vi "stabilizePress_00.vi"() -> ()   [LabVIEW 2011]
uses:
  <vilib>/Platform/TimedLoop/XDataNode/timing_clust.ctl
  <vilib>/Platform/TimedLoop/XDataNode/nitl_modes.ctl
  <vilib>/Platform/TimedLoop/XDataNode/wakeup.ctl
  <vilib>/Platform/TimedLoop/XDataNode/XDataNode.xnode
  <vilib>/Platform/TimedLoop/XDataNode/XDNodeRunTimeDep.lvlib
  <vilib>/Analysis/NI_AALPro.lvlib
panel:
  in  "local when done":bool=TRUE
  out "Best Exponential Fit":dbl[](array[numeric])=[19.840050765406623, 19.861458745604583, 19.86363222245769, 19.863852887909882, 19.863875291296292, 19.863877565833235, 19.86387779675896, 19.86387782020404, 19.86387782258433, 19.863877822825998, 19.863877822850533, 19.863877822853024]
  out "XY Graph":cluster{"Value":dbl[], "Value":dbl[]}[](graph)=[{"Value"=[1.0, 2.0, 3.0, 4.0, 5.0, 6.0, 7.0, 8.0, 9.0, 10.0, 11.0, 12.0], "Value"=[19.84, 19.86, 19.87, 19.87, 19.86, 19.86, 19.86, 19.87, 19.87, 19.86, 19.86, 19.86]}, {"Value"=[1.0, 2.0, 3.0, 4.0, 5.0, 6.0, 7.0, 8.0, 9.0, 10.0, 11.0, 12.0], "Value"=[19.840050765406623, 19.861458745604583, 19.86363222245769, 19.863852887909882, 19.863875291296292, 19.863877565833235, 19.86387779675896, 19.86387782020404, 19.86387782258433, 19.863877822825998, 19.863877822850533, 19.863877822853024]}]
  out "Pfinal (torr)":dbl=19.863877822853304
  out "tune done":bool=TRUE
  in  "max dP step (torr)":dbl=0.1
  out "dP(torr)":dbl
  out "amplitude":dbl=-0.23468810963673434
  out "damping":dbl=-2.287435637167759
  out "tune Setpoint(torr)":dbl=20.0
  in  "t array":dbl[](array[numeric])=[1.0, 2.0, 3.0, 4.0, 5.0, 6.0, 7.0, 8.0, 9.0, 10.0, 11.0, 12.0]
  out "P array":dbl[](array[numeric])=[19.84, 19.86, 19.87, 19.87, 19.86, 19.86, 19.86, 19.87, 19.87, 19.86, 19.86, 19.86]
  out "fit done":bool=TRUE
  in  "tFit(s)":dbl=10.0
  in  "Period (s)":i64=1
  out "Set Point (torr)":dbl=20.0 format="%.2f"
  out "Setpoint Index":string="C"
  out "Setpoint Index control":u16(ring)=2 caption="Setpoint" items=["A", "B", "C", "D"]
  out "first":bool
  out "tStart":dbl=12.0
  in  "time done (s)":dbl
  out "Wait to set":bool
  out "IO error":errorcluster
  in  "stop":bool
  out "P (torr)":dbl=19.86 format="%.2f"
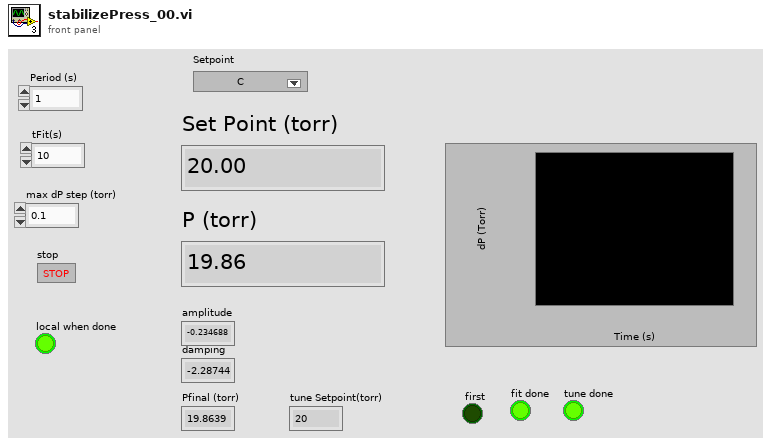
[diagram p1: front panel]
types:
  T1 = typedef "XDNodeRunTimeDep.lvlib/timing_clust.ctl" = cluster{"Expected End [f-1]":u64, "Actual End [f-1]":u64, "Finished Late? [f-1]":bool, "Expected End [i-1]":u64, "Actual End [i-1]":u64, "Finished Late? [i-1]":bool, "Expected Start [i]":u64, "Actual Start [i]":u64, "Expected Start [f]":u64, "Actual Start [f]":u64, "Source Name":string, "Structure Name":string, "Period":i64, "Deadline":i64, "Offset":i64, "Start":i64, "Priority":i32, "Timeout":i32, "Mode":T2, "Wakeup Reason":T3, "Error":errorcluster, "Source Type":string, "Secondary Source Type":string, "Global End Time":u64, "Global Start Time":u64, "Frame Duration":u64, "Iteration Duration":u64, "Assigned CPU":i32, "I/O Scan Engine Mode":u32}
  T2 = typedef "XDNodeRunTimeDep.lvlib/nitl_modes.ctl" = enum32{"No Change", "Process missed periods, maintain original phase", "Discard missed periods, maintain original phase", "Process missed periods, ignore original phase", "Discard missed periods, ignore original phase"}
  T3 = typedef "XDNodeRunTimeDep.lvlib/wakeup.ctl" = enum32{"Normal", "Aborted", "Asynchronous wakeup", "Timing source error", "Timed loop error", "Timeout"}
  T4 = cluster{"amp min":dbl, "amp max":dbl, "damping min":dbl, "damping max":dbl, "offset min":dbl, "offset max":dbl}
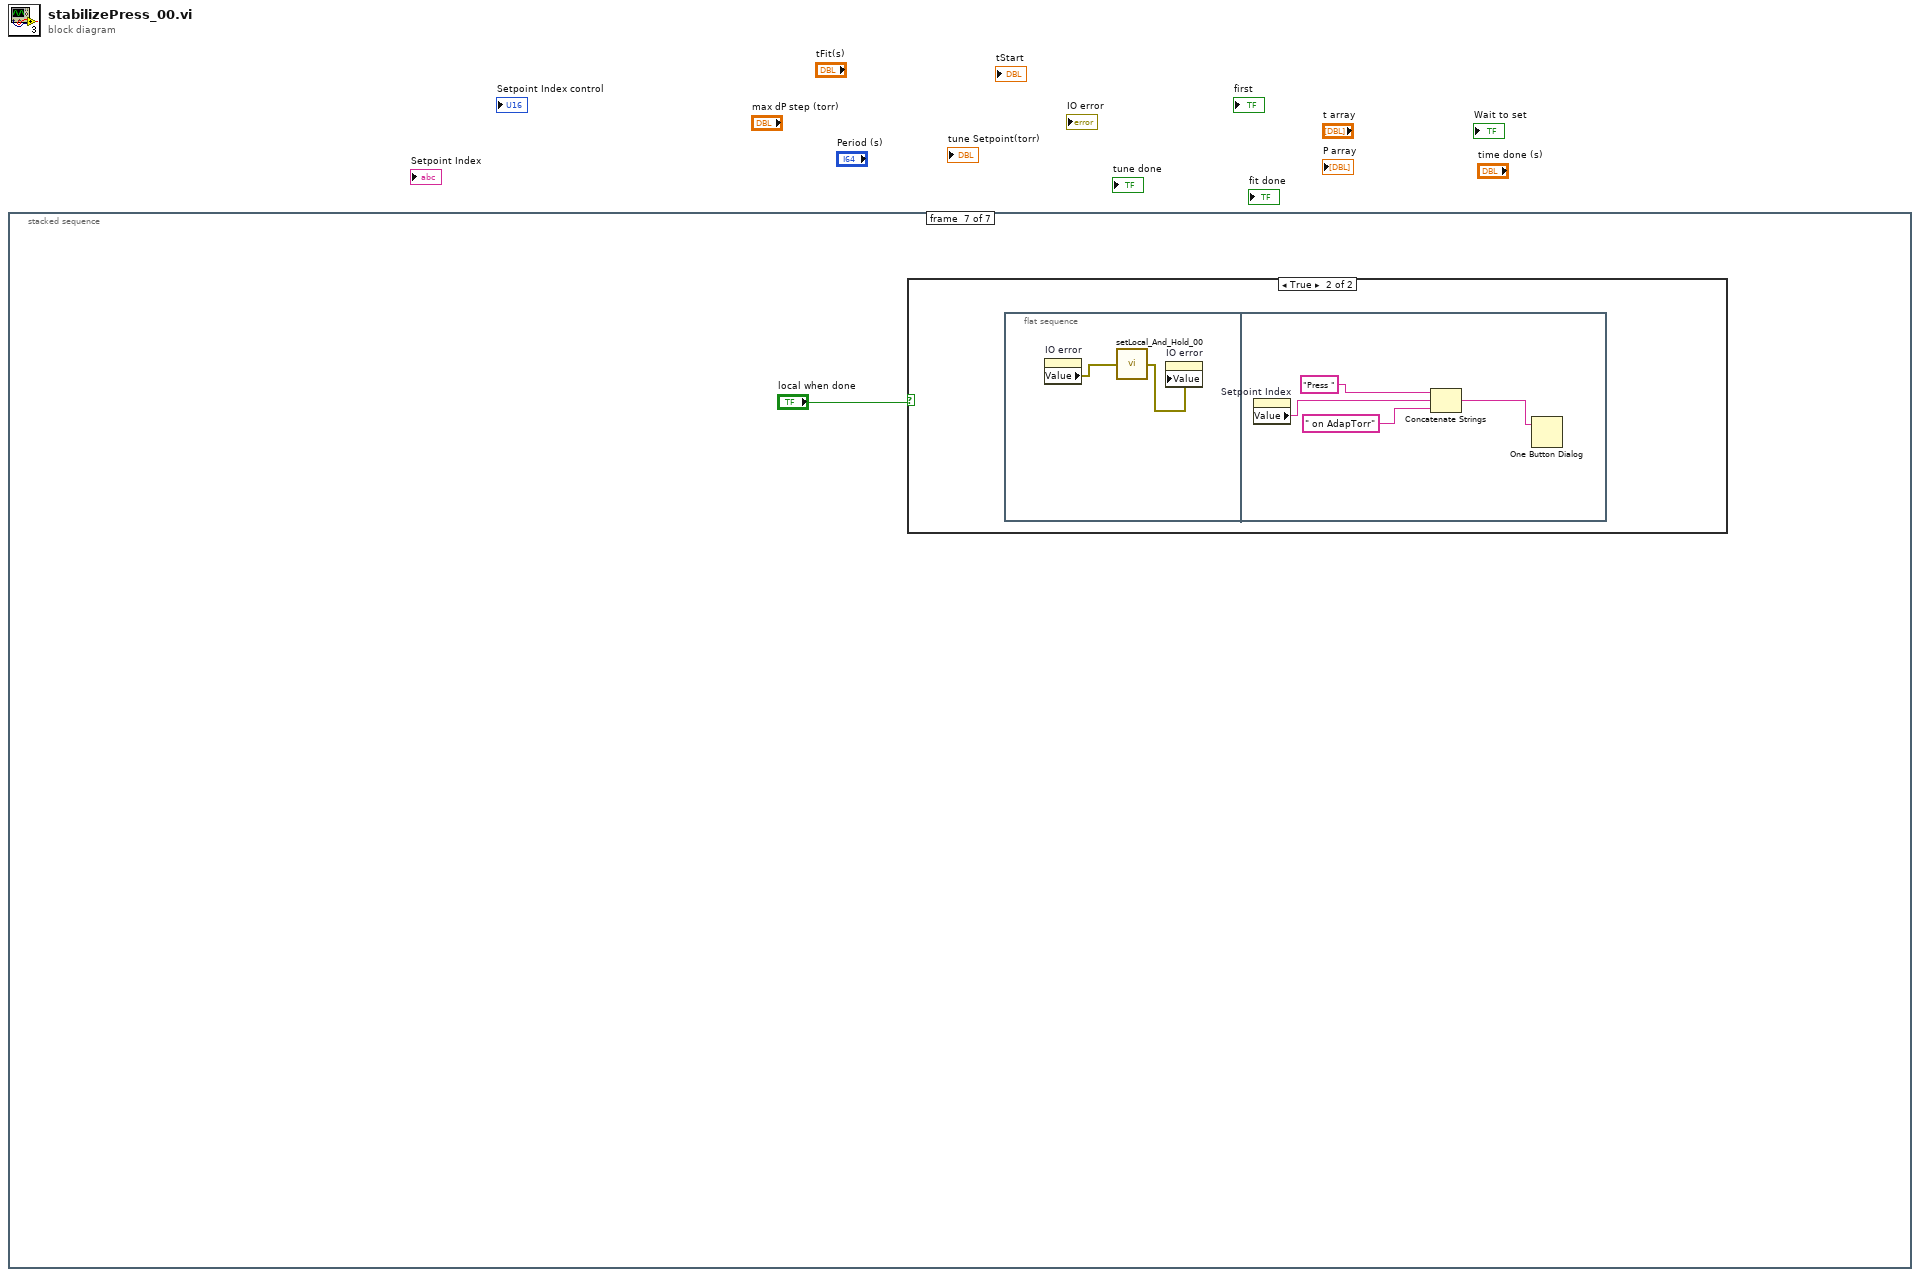
[diagram p0: block diagram]
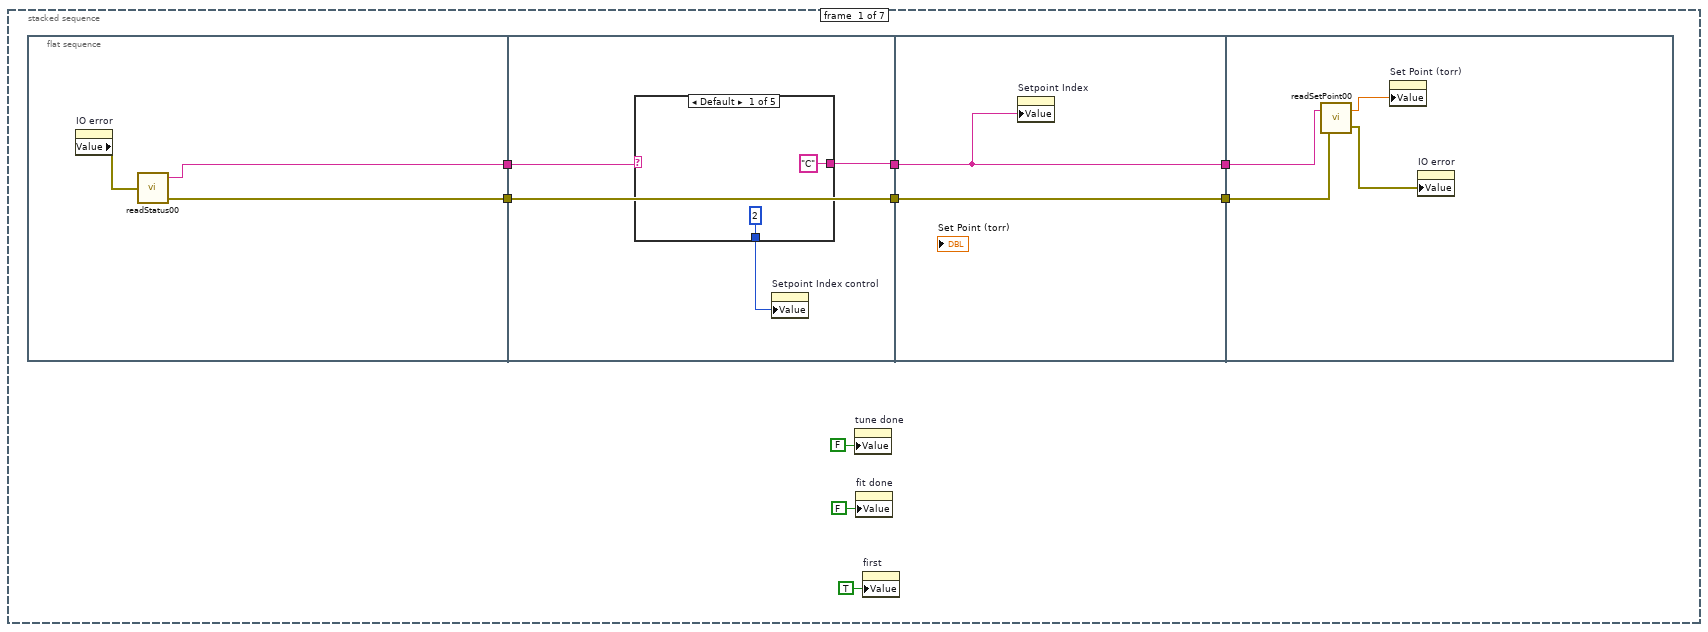
[diagram p2: hidden frame]
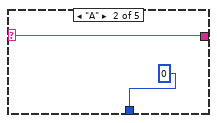
[diagram p3: hidden frame]
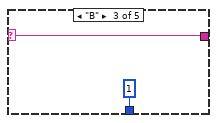
[diagram p4: hidden frame]
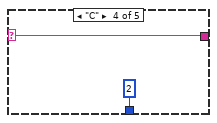
[diagram p5: hidden frame]
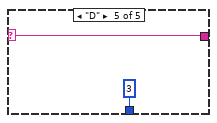
[diagram p6: hidden frame]
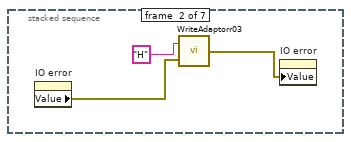
[diagram p7: hidden frame]
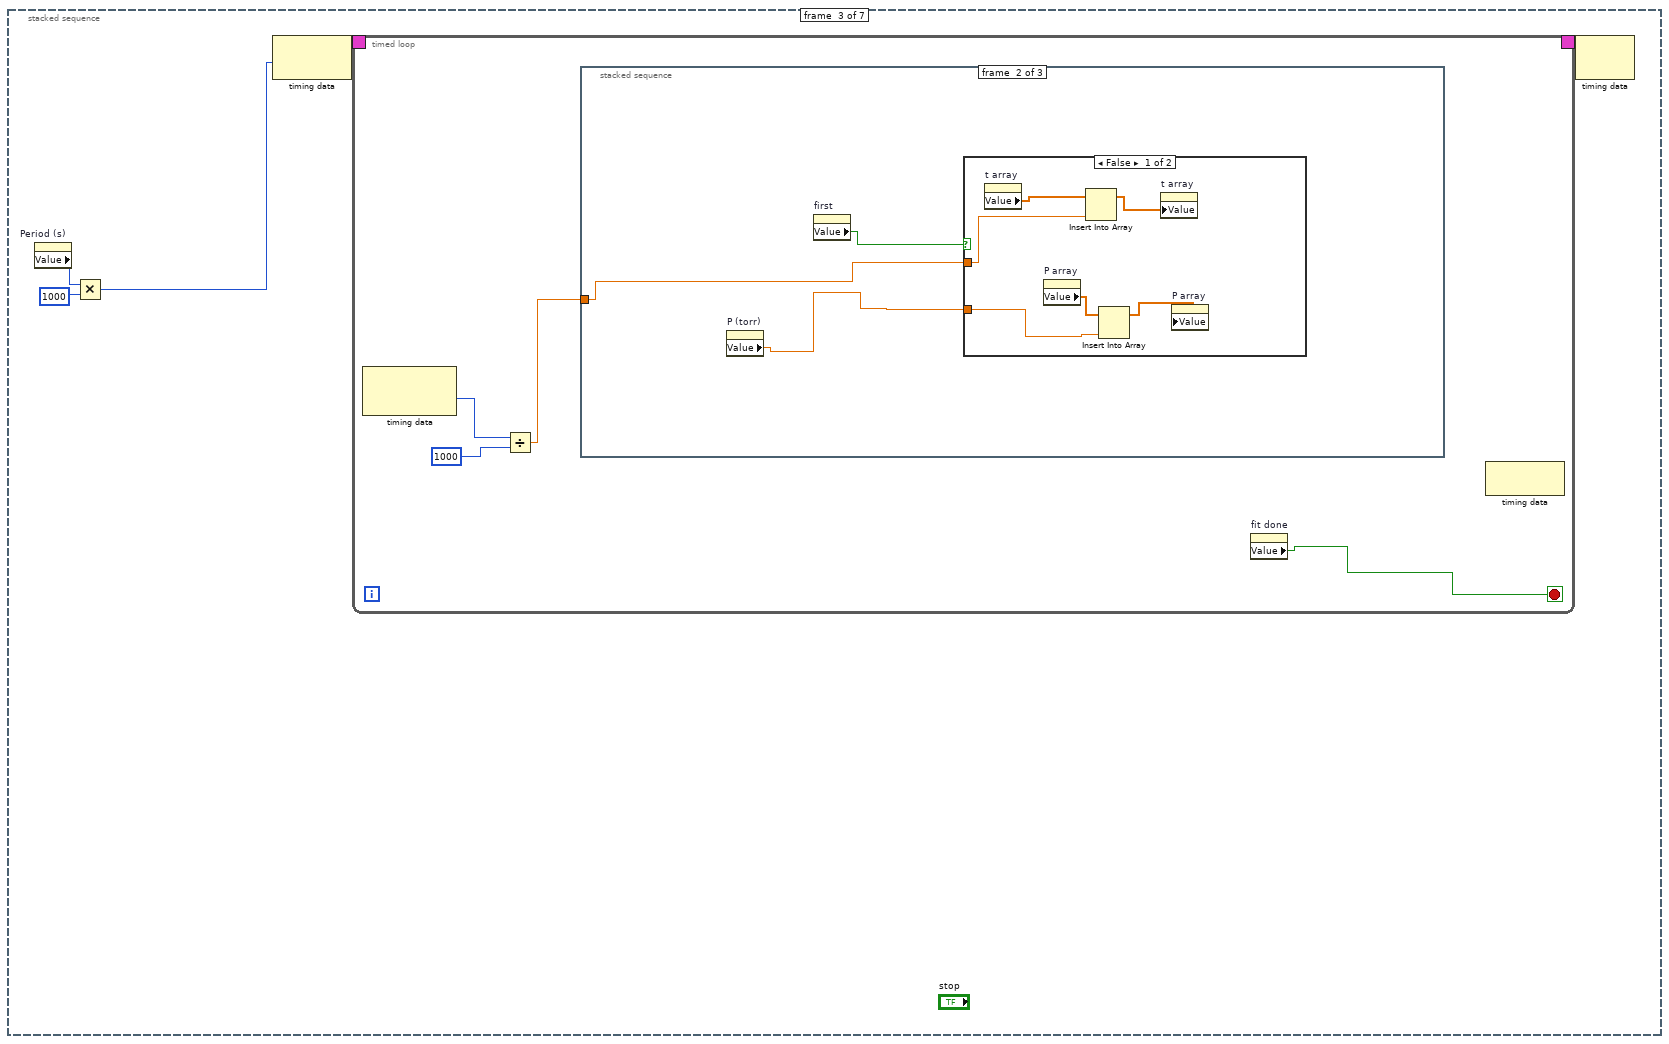
[diagram p8: hidden frame]
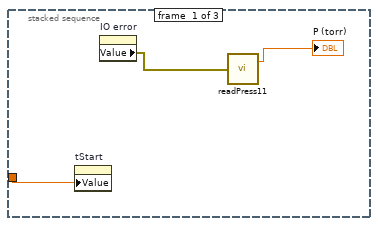
[diagram p9: hidden frame]
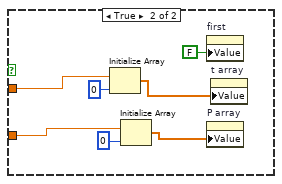
[diagram p10: hidden frame]
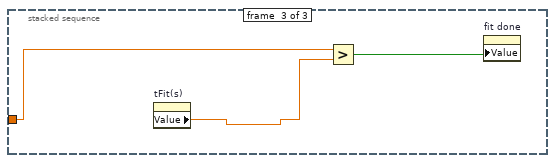
[diagram p11: hidden frame]
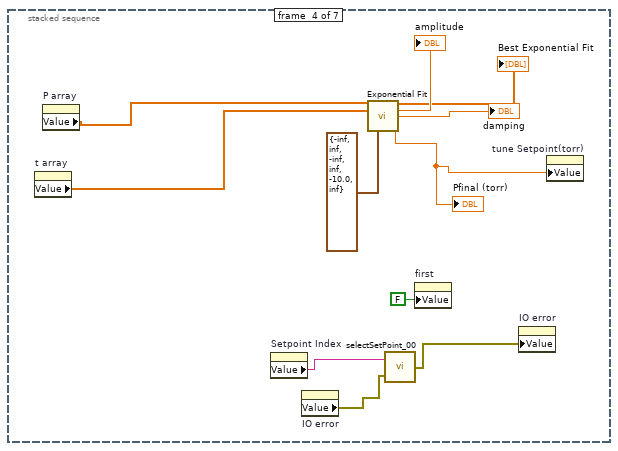
[diagram p12: hidden frame]
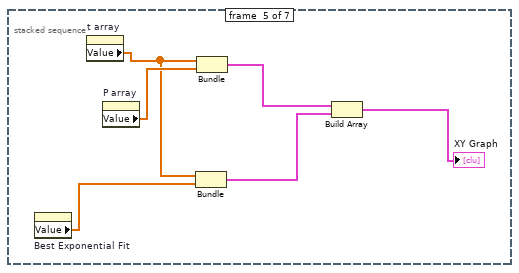
[diagram p13: hidden frame]
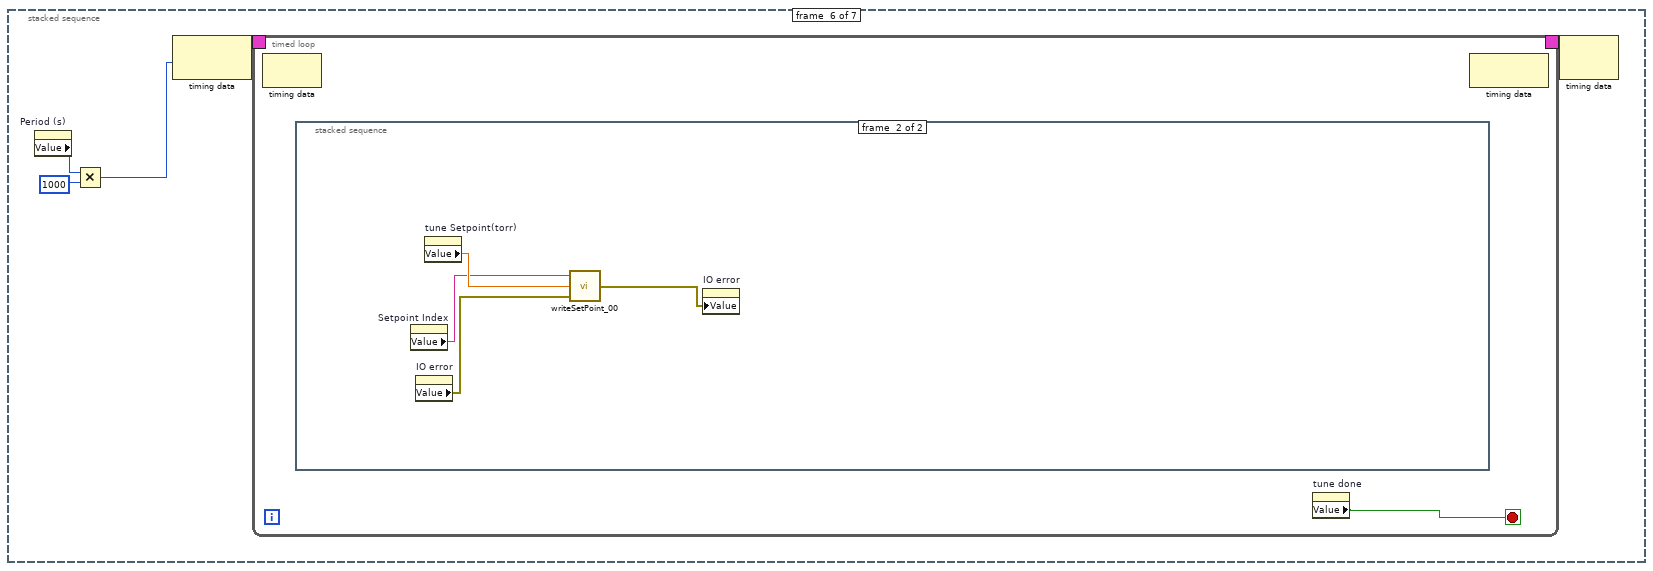
[diagram p14: hidden frame]
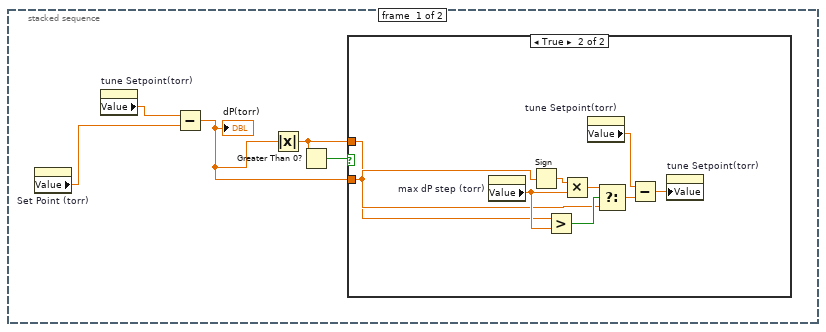
[diagram p15: hidden frame]
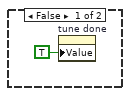
[diagram p16: hidden frame]
diagram:
  n1 = stacked-sequence {
    frame #0 {
      n2 = flat-sequence {
        tunnel: [w11] -> w9
        tunnel: [w10] -> w8
        tunnel: w9 -> [w15]
        tunnel: [w14] -> w7
        tunnel: w8 -> [w16]
        tunnel: [w16] -> w6
        tunnel: w7 -> [w27]
        tunnel: [w27] -> w5
        tunnel: w6 -> [w28]
        tunnel: [w28] -> w4
        tunnel: w5 -> [w32]
        tunnel: w4 -> [w31]
        frame #0 {
          n3 = property on="IO error" class="Clust (strict)"() -> ("Value"=w12:errorcluster)  [unwired: 2 in, 2 out]
          n4 = call "readStatus00.vi"("error in"=w12) -> ("Setpoint"=w11:string, "error out"=w10:errorcluster)  [unwired: 1 out]
        }
        frame #1 {
          n5 = case shown="Default" w15 {
            selector: w15 -> [_ w20 w21 w23 w25]
            tunnel: ["C" w20 w21 w23 w25] -> w14
            tunnel: [u16 2 ("Ring") u16 0 ("Ring") u16 1 ("Ring") u16 2 ("Ring") u16 3 ("Ring")] -> w13
            frame Default {
            }
            frame "A" {
            }
            frame "B" {
            }
            frame "C" {
            }
            frame "D" {
            }
          }
          n6 = property on="Setpoint Index control" class="Ring (strict)"("Value"=w13) -> ()  [unwired: 2 in, 2 out]
        }
        frame #2 {
          n7 = property on="Setpoint Index" class="Str"("Value"=w27) -> ()  [unwired: 2 in, 2 out]
        }
        frame #3 {
          n8 = call "readSetPoint00.vi"("error in"=w31, "Setpoint"=w32) -> ("error out"=w30:errorcluster, "P"=w29:dbl)
          n9 = property on="Set Point (torr)" class="DigNum (strict)"("Value"=w29) -> ()  [unwired: 2 in, 2 out]
          n10 = property on="IO error" class="Clust (strict)"("Value"=w30) -> ()  [unwired: 2 in, 2 out]
        }
      }
      n11 = property on="tune done" class="Bool (strict)"("Value"=FALSE ("tune done")) -> ()  [unwired: 2 in, 2 out]
      n12 = property on="fit done" class="Bool (strict)"("Value"=FALSE ("fit done")) -> ()  [unwired: 2 in, 2 out]
      n13 = property on="first" class="Bool (strict)"("Value"=TRUE ("first")) -> ()  [unwired: 2 in, 2 out]
    }
    frame #1 {
      n14 = property on="IO error" class="Clust (strict)"() -> ("Value"=w34:errorcluster)  [unwired: 2 in, 2 out]
      n15 = call "WriteAdaptorr03.vi"("error in (no error)"=w34, "string to write"="H") -> ("error out"=w33:errorcluster)
      n16 = property on="IO error" class="Clust (strict)"("Value"=w33) -> ()  [unwired: 2 in, 2 out]
    }
    frame #2 {
      n17 = property on="Period (s)" class="DigNum (strict)"() -> ("Value"=w37:i64)  [unwired: 2 in, 2 out]
      n18 = Multiply(x=w37, y=u32 1000) -> (x*y=w36:i64)
      n19 = node-c288(w36) -> (w40:T1)
      n20 = timed-loop {
        timing: w40 -> [_]
        timing-out: [_] -> w39
        stop <- w41 stop-if-true
        n21 = node-c288() -> (w44:i64)  [unwired: 1 in, 1 out]
        n22 = Divide(x=w44, y=i64 1000) -> (x/y=w42:dbl)
        n23 = stacked-sequence {
          tunnel: w42 -> [w47 w48 w66]
          frame #0 {
            n24 = property on="tStart" class="DigNum (strict)"("Value"=w47) -> ()  [unwired: 2 in, 2 out]
            n25 = property on="IO error" class="Clust (strict)"() -> ("Value"=w45:errorcluster)  [unwired: 2 in, 2 out]
            n26 = call "readPress11.vi"("error in"=w45) -> ("P"=→"P (torr)":dbl)  [unwired: 1 out]
          }
          frame #1 {
            n27 = property on="P (torr)" class="DigNum (strict)"() -> ("Value"=w49:dbl)  [unwired: 2 in, 2 out]
            n28 = property on="first" class="Bool (strict)"() -> ("Value"=w50:bool)  [unwired: 2 in, 2 out]
            n29 = case shown="False" w50 {
              tunnel: w49 -> [w56 w62]
              tunnel: w48 -> [w53 w60]
              frame False {
                n30 = property on="t array" class="Arr (strict)"() -> ("Value"=w52:dbl[])  [unwired: 2 in, 2 out]
                n31 = property on="P array" class="Arr (strict)"() -> ("Value"=w54:dbl[])  [unwired: 2 in, 2 out]
                n32 = Insert Into Array(array=w52, new element=w53) -> (w51:dbl[])  [unwired: 1 in]
                n33 = Insert Into Array(array=w54, new element=w56) -> (w55:dbl[])  [unwired: 1 in]
                n34 = property on="t array" class="Arr (strict)"("Value"=w51) -> ()  [unwired: 2 in, 2 out]
                n35 = property on="P array" class="Arr (strict)"("Value"=w55) -> ()  [unwired: 2 in, 2 out]
              }
              frame True {
                n36 = Initialize Array(w60, 0 ("dimension size")) -> (w57:dbl[])
                n37 = Initialize Array(w62, 0 ("dimension size")) -> (w58:dbl[])
                n38 = property on="first" class="Bool (strict)"("Value"=FALSE ("first")) -> ()  [unwired: 2 in, 2 out]
                n39 = property on="P array" class="Arr (strict)"("Value"=w58) -> ()  [unwired: 2 in, 2 out]
                n40 = property on="t array" class="Arr (strict)"("Value"=w57) -> ()  [unwired: 2 in, 2 out]
              }
            }
          }
          frame #2 {
            n41 = property on="tFit(s)" class="DigNum (strict)"() -> ("Value"=w64:dbl)  [unwired: 2 in, 2 out]
            n42 = Greater?(x=w66, y=w64) -> (0:w65:bool)
            n43 = property on="fit done" class="Bool (strict)"("Value"=w65) -> ()  [unwired: 2 in, 2 out]
          }
        }
        n44 = property on="fit done" class="Bool (strict)"() -> ("Value"=w41:bool)  [unwired: 2 in, 2 out]
        n45 = node-c288() -> ()  [unwired: 1 in, 1 out]
      }
      n46 = node-c288(w39) -> ()  [unwired: 1 out]
    }
    frame #3 {
      n47 = property on="t array" class="Arr (strict)"() -> ("Value"=w83:dbl[])  [unwired: 2 in, 2 out]
      n48 = property on="P array" class="Arr (strict)"() -> ("Value"=w84:dbl[])  [unwired: 2 in, 2 out]
      n49 = property on="Setpoint Index" class="Str"() -> ("Value"=w78:string)  [unwired: 2 in, 2 out]
      n50 = property on="IO error" class="Clust (strict)"() -> ("Value"=w77:errorcluster)  [unwired: 2 in, 2 out]
      n51 = call <vilib>:"Exponential Fit.vi"("Y"=w84, "X"=w83, "parameter bounds"=T4 {"amp min"=-inf, "amp max"=inf, "damping min"=-inf, "damping max"=inf, "offset min"=-10.0, "offset max"=inf}) -> ("Best Exponential Fit"=→"Best Exponential Fit":dbl[], "amplitude"=→"amplitude":dbl, "damping"=→"damping":dbl, "offset"=w80:dbl)  [unwired: 7 in, 2 out]
      "Pfinal (torr)" <- w80
      n52 = call "selectSetPoint_00.vi"("error in"=w77, "Setpoint"=w78) -> ("error out"=w76:errorcluster)
      n53 = property on="first" class="Bool (strict)"("Value"=FALSE ("first")) -> ()  [unwired: 2 in, 2 out]
      n54 = property on="IO error" class="Clust (strict)"("Value"=w76) -> ()  [unwired: 2 in, 2 out]
      n55 = property on="tune Setpoint(torr)" class="DigNum (strict)"("Value"=w80) -> ()  [unwired: 2 in, 2 out]
    }
    frame #4 {
      n56 = property on="Best Exponential Fit" class="Arr (strict)"() -> ("Value"=w88:dbl[])  [unwired: 2 in, 2 out]
      n57 = property on="t array" class="Arr (strict)"() -> ("Value"=w89:dbl[])  [unwired: 2 in, 2 out]
      n58 = property on="P array" class="Arr (strict)"() -> ("Value"=w90:dbl[])  [unwired: 2 in, 2 out]
      n59 = Bundle "Bundle"("Value"=w89, "Value"=w88) -> (w86:cluster{"Value":dbl[], "Value":dbl[]})  [unwired: 1 in]
      n60 = Bundle "Bundle"("Value"=w89, "Value"=w90) -> (w87:cluster{"Value":dbl[], "Value":dbl[]})  [unwired: 1 in]
      n61 = Build Array "Build Array"(w87, w86) -> (→"XY Graph":cluster{"Value":dbl[], "Value":dbl[]}[])
    }
    frame #5 {
      n62 = property on="Period (s)" class="DigNum (strict)"() -> ("Value"=w93:i64)  [unwired: 2 in, 2 out]
      n63 = Multiply(x=w93, y=u32 1000) -> (x*y=w91:i64)
      n64 = node-c288(w91) -> (w95:T1)
      n65 = timed-loop {
        timing: w95 -> [_]
        timing-out: [_] -> w94
        stop <- w96 stop-if-true
        n66 = node-c288() -> ()  [unwired: 1 in, 1 out]
        n67 = stacked-sequence {
          frame #0 {
            n68 = property on="Set Point (torr)" class="DigNum (strict)"() -> ("Value"=w101:dbl)  [unwired: 2 in, 2 out]
            n69 = property on="tune Setpoint(torr)" class="DigNum (strict)"() -> ("Value"=w100:dbl)  [unwired: 2 in, 2 out]
            n70 = Subtract(x=w100, y=w101) -> (x-y=w99:dbl)
            "dP(torr)" <- w99
            n71 = Absolute Value(x=w99) -> (abs(x)=w98:dbl)
            n72 = Greater Than 0?(x=w98) -> (x > 0?=w97:bool)
            n73 = case shown="True" w97 {
              tunnel: w99 -> [_ w107]
              tunnel: w98 -> [_ w103]
              frame False {
                n74 = property on="tune done" class="Bool (strict)"("Value"=TRUE ("tune done")) -> ()  [unwired: 2 in, 2 out]
              }
              frame True {
                n75 = property on="max dP step (torr)" class="DigNum (strict)"() -> ("Value"=w109:dbl)  [unwired: 2 in, 2 out]
                n76 = Sign(1:w107) -> (0:w110:dbl)
                n77 = Greater?(x=w103, y=w109) -> (0:w111:bool)
                n78 = Multiply(x=w110, y=w109) -> (x*y=w108:dbl)
                n79 = property on="tune Setpoint(torr)" class="DigNum (strict)"() -> ("Value"=w106:dbl)  [unwired: 2 in, 2 out]
                n80 = Select(t=w108, s=w111, f=w107) -> (s? t:f=w105:dbl)
                n81 = Subtract(x=w106, y=w105) -> (x-y=w104:dbl)
                n82 = property on="tune Setpoint(torr)" class="DigNum (strict)"("Value"=w104) -> ()  [unwired: 2 in, 2 out]
              }
            }
          }
          frame #1 {
            n83 = property on="Setpoint Index" class="Str"() -> ("Value"=w114:string)  [unwired: 2 in, 2 out]
            n84 = property on="IO error" class="Clust (strict)"() -> ("Value"=w113:errorcluster)  [unwired: 2 in, 2 out]
            n85 = property on="tune Setpoint(torr)" class="DigNum (strict)"() -> ("Value"=w115:dbl)  [unwired: 2 in, 2 out]
            n86 = call "writeSetPoint_00.vi"("error in"=w113, "P (Torr)"=w115, "Setpoint"=w114) -> ("error out"=w112:errorcluster)
            n87 = property on="IO error" class="Clust (strict)"("Value"=w112) -> ()  [unwired: 2 in, 2 out]
          }
        }
        n88 = property on="tune done" class="Bool (strict)"() -> ("Value"=w96:bool)  [unwired: 2 in, 2 out]
        n89 = node-c288() -> ()  [unwired: 1 in, 1 out]
      }
      n90 = node-c288(w94) -> ()  [unwired: 1 out]
    }
    frame #6 {
      n91 = case shown="True" "local when done" {
        frame False {
        }
        frame True {
          n92 = flat-sequence {
            frame #0 {
              n93 = property on="IO error" class="Clust (strict)"() -> ("Value"=w124:errorcluster)  [unwired: 2 in, 2 out]
              n94 = call "setLocal_And_Hold_00.vi"("error in (no error)"=w124) -> ("error out"=w123:errorcluster)
              n95 = property on="IO error" class="Clust (strict)"("Value"=w123) -> ()  [unwired: 2 in, 2 out]
            }
            frame #1 {
              n96 = property on="Setpoint Index" class="Str"() -> ("Value"=w126:string)  [unwired: 2 in, 2 out]
              n97 = Concatenate Strings("Press ", w126, " on AdapTorr") -> (w125:string)
              n98 = One Button Dialog(message=w125) -> ()  [unwired: 1 in, 1 out]
            }
          }
        }
      }
    }
  }
